vi "Emballage_BDD_lecture_Table_Correspondance_avec_index.vi"(6 "ID_ARTICLE":string, 8 "entrée d'erreur (pas d'erreur)":errorcluster, 9 "ID_ARTICLE?":bool, 10 "Piece_Scanne":string, 11 "ligne_Table_correspondance":string[](array[string])) -> (0 "sortie d'erreur":errorcluster, 2 "Table_BDD":string, 3 "info":string)   [LabVIEW 2020]
panel:
  out "champs_valve":string[](array[string])
  out "valeur_condition":string[](array[string])
  out "champs_condition":string[](array[string])
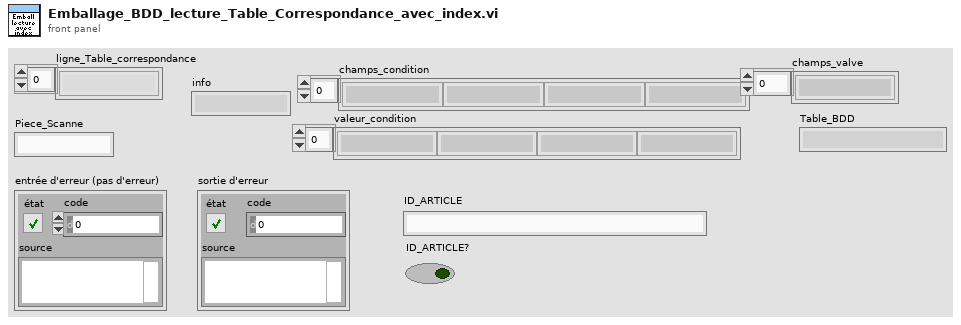
[diagram p1: front panel]
types:
  T1 = typedef "Emballage_Index_correspondance.ctl" = cluster{"Index_CHAMP_RESULTAT":i32, "Index_TABLE_BDD":i32, "Index_CHAMP_ORDRE":i32, "Index_VALEUR_RESULTAT":i32, "Index_FAMILLE_VALVE":i32, "Index_NO_VALVE":i32, "Index_CHAMPS_CONDITION":i32, "Index_VALEUR_CONDITION":i32}
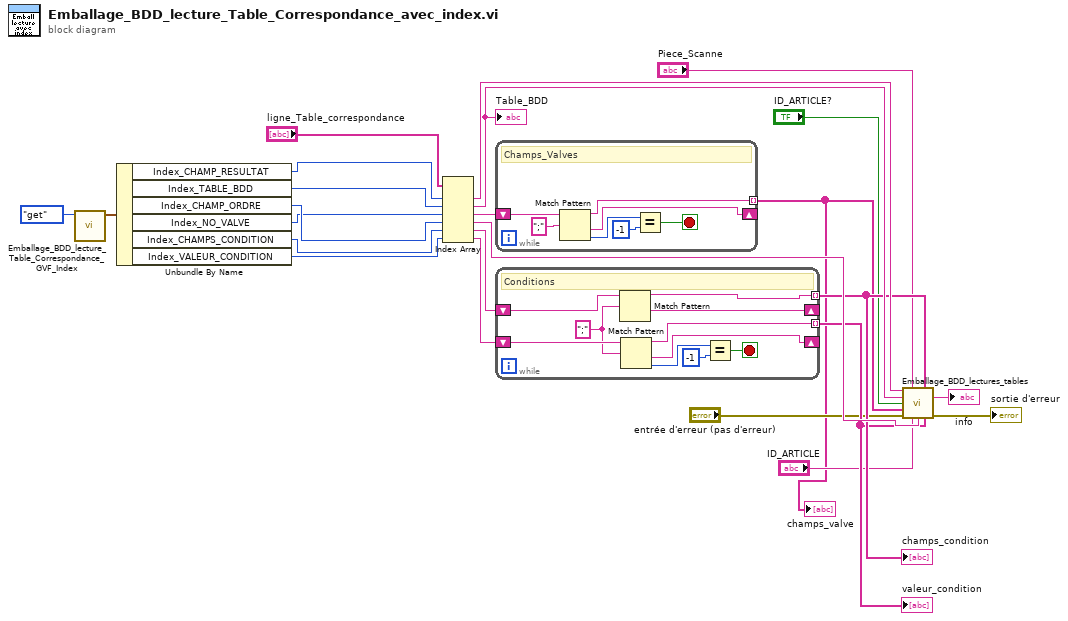
[diagram p0: block diagram]
diagram:
  n1 = call "Emballage_BDD_lecture_Table_Correspondance_GVF_Index.vi"("Énum"=enum16{"get", "set"}."get") -> ("Cluster_index_champs_correspondance"=w20:T1)  [unwired: 10 in]
  n2 = Unbundle By Name(w20) -> ("Index_CHAMP_RESULTAT"=w21:i32, "Index_TABLE_BDD"=w22:i32, "Index_CHAMP_ORDRE"=w24:i32, "Index_NO_VALVE"=w23:i32, "Index_CHAMPS_CONDITION"=w13:i32, "Index_VALEUR_CONDITION"=w12:i32)
  n3 = Index Array(array="ligne_Table_correspondance", index #1=w21, index #2=w22, index #3=w23, index #4=w24, index #5=w13, index #6=w12) -> (element #1=w17:string, element #2=w18:string, element #3=w2:string, element #4=w19:string, element #5=w10:string, element #6=w11:string)
  "Table_BDD" <- w18
  n4 = while {
    shift-right: [w29] -> _
    shift-left: w2 -> [w31]
    tunnel: [w25] -> w1 mode=indexing
    stop <- w28 stop-if-true
    # "Champs_Valves"
    n5 = Match Pattern(string=w31, regular expression=";" ("expression régulière")) -> (before substring=w25:string, after substring=w29:string, offset past match=w27:i32)  [unwired: 1 in, 1 out]
    n6 = Equal?(x=w27, y=-1) -> (x = y?=w28:bool)
  }
  "champs_valve" <- w1
  n7 = while {
    shift-right: [w38] -> _
    shift-left: w10 -> [w41]
    shift-right: [w37] -> _
    shift-left: w11 -> [w40]
    tunnel: [w33] -> w9 mode=indexing
    tunnel: [w32] -> w8 mode=indexing
    stop <- w36 stop-if-true
    w39 = ";" ("expression régulière")
    # "Conditions"
    n8 = Match Pattern(string=w41, regular expression=w39) -> (before substring=w33:string, after substring=w38:string)  [unwired: 1 in, 2 out]
    n9 = Match Pattern(string=w40, regular expression=w39) -> (before substring=w32:string, after substring=w37:string, offset past match=w35:i32)  [unwired: 1 in, 1 out]
    n10 = Equal?(x=w35, y=-1) -> (x = y?=w36:bool)
  }
  "champs_condition" <- w9
  "valeur_condition" <- w8
  n11 = call "Emballage_BDD_lectures_tables.vi"("Champ_resultat"=w17, "num_piece"="Piece_Scanne", "Champs-condition"=w9, "Table_BDD"=w18, "ID_ARTICLE?"="ID_ARTICLE?", "VALVE"=w1, "entrée d'erreur (pas d'erreur)"="entrée d'erreur (pas d'erreur)", "ID_ARTICLE"="ID_ARTICLE", "Champ_ordre"=w19, "valeur_condition"=w8) -> ("info"=→"info":string, "sortie d'erreur"=→"sortie d'erreur":errorcluster)  [unwired: 3 in, 1 out]
